vi "4_8.vi"() -> ()   [LabVIEW 2020]
uses:
  <vilib>/numeric/Random Number (Range) I64.vi
  <vilib>/numeric/sub_Random U32.vi
panel:
  in  "OK Button":bool
  out "output array":i64[][](array[numeric])
  in  "K":i64
  in  "Num":i32
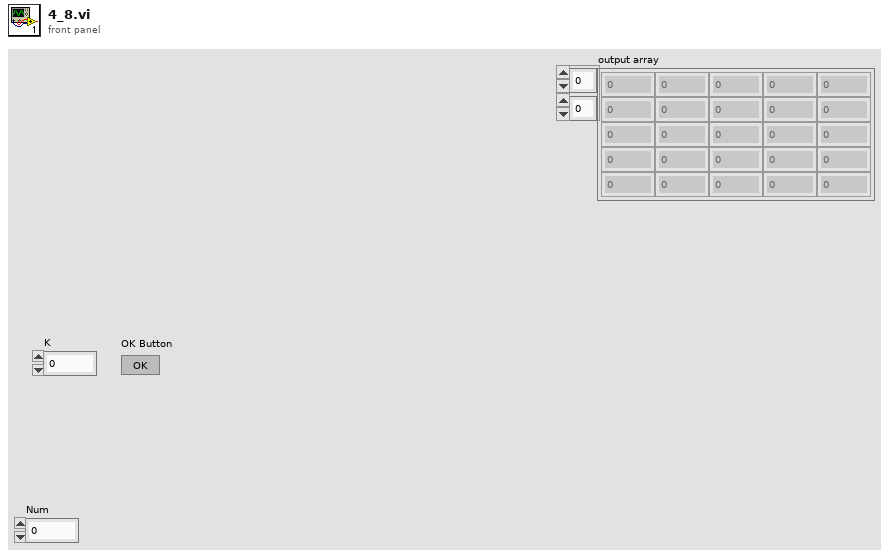
[diagram p1: front panel]
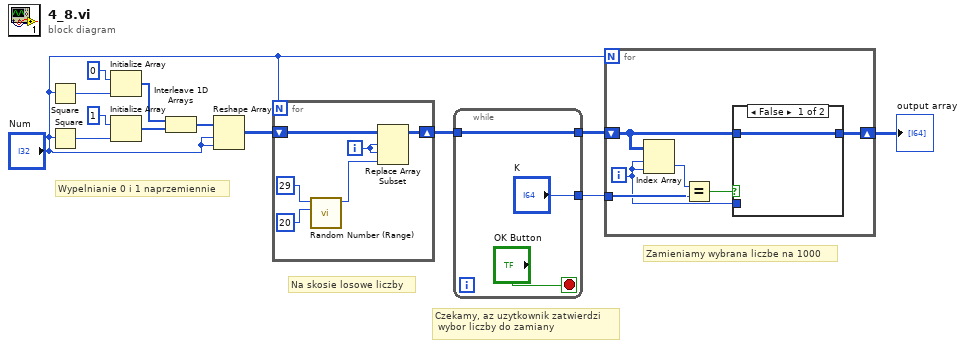
[diagram p0: block diagram]
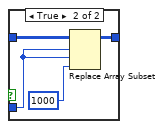
[diagram p2: hidden frame]
diagram:
  # "Zamieniamy wybrana liczbe na 1000"
  # "Czekamy, az uzytkownik zatwierdzi\n wybor liczby do zamiany"
  # "Na skosie losowe liczby"
  # "Wypelnianie 0 i 1 naprzemiennie"
  n1 = Square(x="Num") -> (x^2=w8:i32)
  n2 = Square(x="Num") -> (x^2=w7:i32)
  n3 = Initialize Array(i64 0 ("element"), w8) -> (w11:i64[])
  n4 = Initialize Array(i64 1 ("element"), w7) -> (w10:i64[])
  n5 = Interleave 1D Arrays(w11, w10) -> (w9:i64[])
  n6 = Reshape Array(w9, "Num", "Num") -> (w6:i64[][])
  n7 = for {
    N: "Num" -> [_]
    shift-right: [w14] -> w3
    shift-left: w6 -> [w17]
    i -> [w16]
    n8 = call-poly <vilib>:"Random Number (Range).vi"("lower bound (-100)"=i64 20 ("lower bound (0)"), "upper bound (100)"=i64 29) -> ("number"=w15:i64)  [unwired: 9 in]
    n9 = Replace Array Subset(array=w17, new element=w15, index (row)=w16, index (col)=w16) -> (w14:i64[][])
  }
  n10 = while {
    tunnel: [w22] -> w4
    tunnel: w3 -> [w22]
    tunnel: ["K"] -> w1
    stop <- "OK Button" stop-if-true
  }
  n11 = for {
    N: "Num" -> [_]
    tunnel: w1 -> [w27]
    shift-right: [w23] -> w5
    shift-left: w4 -> [w25]
    i -> [w24]
    n12 = Index Array(array=w25, index (row)=w24, index (col)=w24) -> (element=w28:i64)
    n13 = Equal?(x=w28, y=w27) -> (x = y?=w26:bool)
    n14 = case shown="False" w26 {
      tunnel: w25 -> [w29 w33]
      tunnel: w24 -> [_ w32]
      tunnel: [w29 w30] -> w23
      frame False {
      }
      frame True {
        n15 = Replace Array Subset(array=w33, new element=i64 1000 ("new element/subarray"), index (row)=w32, index (col)=w32) -> (w30:i64[][])
      }
    }
  }
  "output array" <- w5
